vi "Report Read Error.vi"(8 "error in (no error)":errorcluster, 11 "Success":bool) -> (0 "error out":errorcluster)   [LabVIEW 2017]
uses:
  <vilib>/Rock Robotics/Network Tables/NT Globals.vi
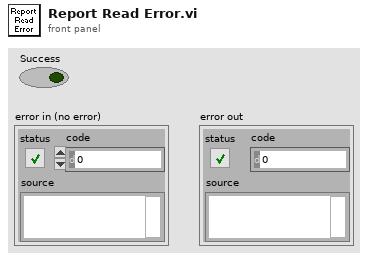
[diagram p1: front panel]
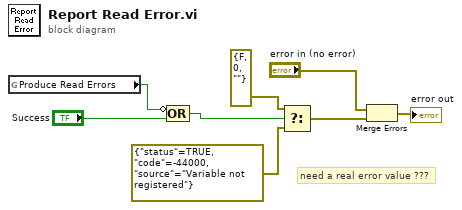
[diagram p0: block diagram]
diagram:
  # "need a real error value ???"
  n1 = global read "NT Globals.vi" "Produce Read Errors"() -> (w1:bool)
  n2 = Compound Arithmetic op=OR(invert w1, "Success") -> (w2:bool)
  n3 = Select(t=errorcluster {"status"=FALSE, "code"=0, "source"=""} ("error in (no error)"), s=w2, f=errorcluster {"status"=TRUE, "code"=-44000, "source"="Variable not registered"} ("error in (no error)")) -> (s? t:f=w4:errorcluster)
  n4 = Merge Errors("error in (no error)", w4) -> (→"error out":errorcluster)
